vi "Build Scheduled Message Configuration(1553).vi"(9 "skip (F)":bool, 10 "singleShot (F)":bool, 11 "messageIDRef":i32) -> (3 "1553 Scheduled Message Configuration out":T1)   [LabVIEW 2020, in "Ballard_1553_Hardware_ni.lvlib"]
uses:
  Ballard_1553_Hardware_ni.lvlib
  _typedefs/schedItem1553_type.ctl
  _typedefs/frame_entry_type.ctl
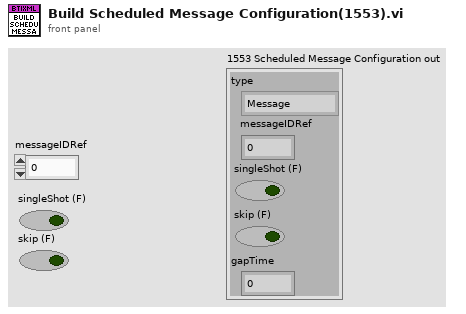
[diagram p1: front panel]
types:
  T1 = typedef "Ballard_1553_Hardware_ni.lvlib/schedItem1553_type.ctl" = cluster{"type":T2, "messageIDRef":i32, "singleShot (F)":bool, "skip (F)":bool, "gapTime":dbl}
  T2 = typedef "Ballard_1553_Hardware_ni.lvlib/frame_entry_type.ctl" = enum16{"Message", "Gap", "Pulse", "Log", "Pause", "Restart", "Halt"}
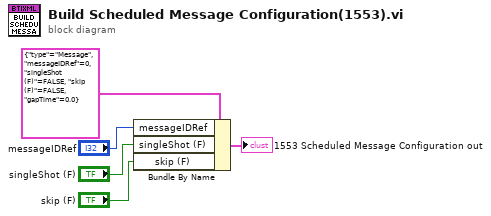
[diagram p0: block diagram]
diagram:
  n1 = Bundle By Name(cluster=T1 {"type"=enum."Message", "messageIDRef"=0, "singleShot (F)"=FALSE, "skip (F)"=FALSE, "gapTime"=0.0} ("Enum"), "messageIDRef"="messageIDRef", "singleShot (F)"="singleShot (F)", "skip (F)"="skip (F)") -> (→"1553 Scheduled Message Configuration out":T1)
